vi "imaqio_FindDevice2.vi"(8 "error in (no error)":errorcluster, 11 "Resource In":T1) -> (0 "error out":errorcluster, 2 "All Resources":T1[](array[typedef]), 3 "Resource Out":T1)   [LabVIEW 2017]
uses:
  <vilib>/userdefined/High Color/nirio_resource_hc.ctl
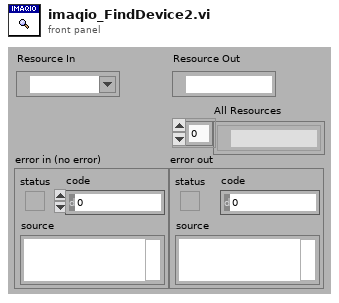
[diagram p1: front panel]
types:
  T1 = typedef "nirio_resource_hc.ctl" = tag
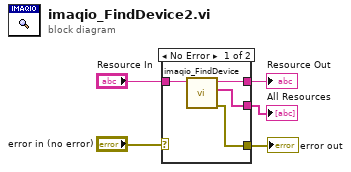
[diagram p0: block diagram]
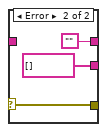
[diagram p2: hidden frame]
diagram:
  n1 = case shown="No Error" "error in (no error)" {
    selector: "error in (no error)" -> [_ w12]
    tunnel: "Resource In" -> [w9 _]
    tunnel: [w8 ""] -> w3
    tunnel: [w7 w12] -> w2
    tunnel: [w6 string[] [] ("Found Devices")] -> w1
    frame No Error {
      n2 = call <vilib>:"imaqio_FindDevice.vi"("Resource In"=w9) -> ("error out"=w7:errorcluster, "All Resources"=w6:string[], "Resource Out"=w8:string)  [unwired: 1 in, 7 out]
    }
    frame Error {
    }
  }
  "error out" <- w2
  "Resource Out" <- w3
  "All Resources" <- w1
